vi "Create.vi"(8 "error in (no error)":errorcluster, 10 "LabVIEW Build":T1, 11 "Description":string) -> (0 "error out":errorcluster, 3 "LabVIEW Build out":refnum<class "LabVIEW Build.lvclass">)   [LabVIEW 2014, in "LabVIEW Build.lvclass"]
uses:
  LabVIEW Build.lvclass
  Shared/Controls/LabVIEW Build - STYP.ctl
  Build Job/Build Job.lvclass/Build Job.ctl
  LabVIEW Build.lvclass/LabVIEW Build.ctl
  Build Job/Write Script Job Name.vi
  Build Job/Write Job Description.vi
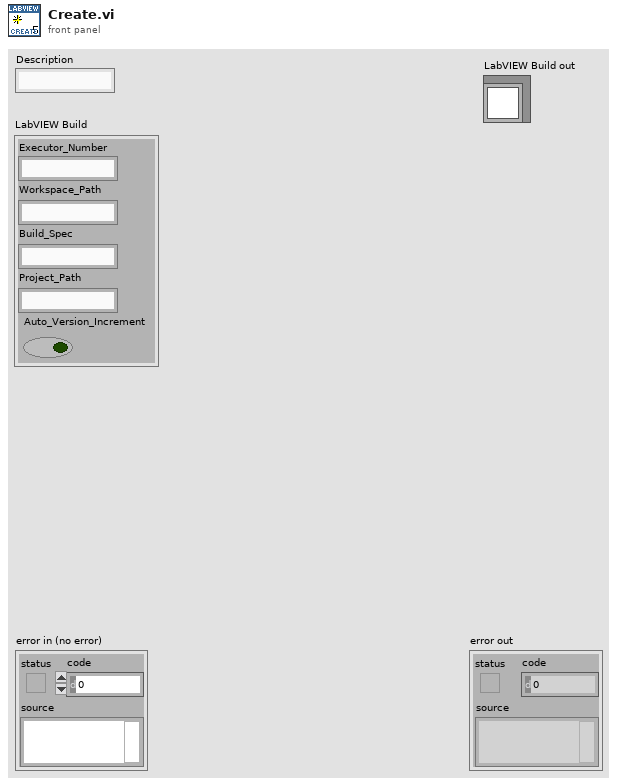
[diagram p1: front panel]
types:
  T1 = typedef "LabVIEW Build - STYP.ctl" = cluster{"Executor_Number":string, "Workspace_Path":string, "Build_Spec":string, "Project_Path":string, "Auto_Version_Increment":bool}
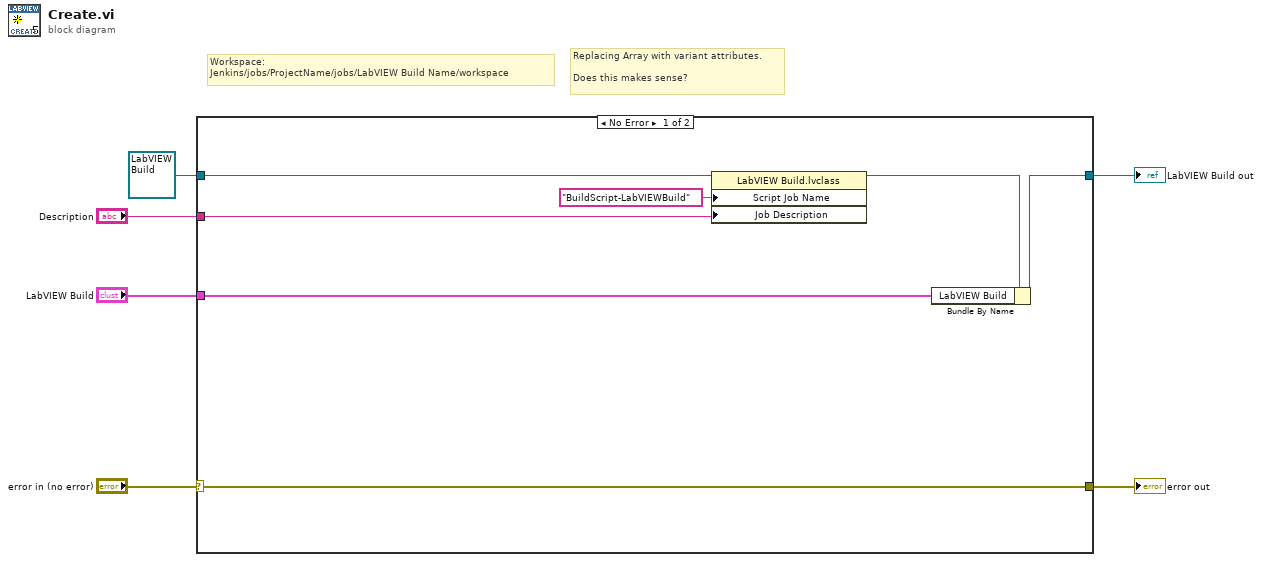
[diagram p0: block diagram]
diagram:
  # "Replacing Array with variant attributes.  \n\nDoes this makes sense?"
  # "Workspace:\nJenkins/jobs/ProjectName/jobs/LabVIEW Build Name/workspace"
  n1 = case shown="No Error" "error in (no error)" {
    selector: "error in (no error)" -> [w8 w15]
    tunnel: [w8 w15] -> w5
    tunnel: [w9 w14] -> w3
    tunnel: refnum<class "LabVIEW Build.lvclass"> refnum ("LabVIEW Build in") -> [w13 w14]
    tunnel: "Description" -> [w7 _]
    tunnel: "LabVIEW Build" -> [w11 _]
    frame No Error {
      n2 = property class="LabVIEW Build.lvclass"(reference=w13, "Script Job Name"="BuildScript-LabVIEWBuild", "Job Description"=w7) -> (reference out=w10:refnum<class "LabVIEW Build.lvclass">)  [unwired: 1 in, 1 out]
      n3 = Bundle By Name(cluster=w10, "LabVIEW Build"=w11) -> (w9:refnum<class "LabVIEW Build.lvclass">)
    }
    frame Error {
    }
  }
  "error out" <- w5
  "LabVIEW Build out" <- w3
